vi "SetScanParameters.vi"(0 "Scan Parameters Cluster":T1={"Lines"=-2147483648, "Columns"=-2147483648, "X Range "=-inf, "Y Range "=-inf, "Pixel Size"=-inf, "Origin X"=-inf, "Origin Y"=-inf, "Rotation"=-inf, "Sample Time"=-inf} {"Sample Time" format="%#_g µs"; "Rotation" format="%#_g deg"; "Origin Y" format="%#_g nm"; "Origin X" format="%#_g nm"; "Pixel Size" format="%#_g nm"; "Y Range" format="%#_g nm"; "X Range" format="%#_g nm"; "Columns" max=250; "Lines" max=250}, 5 "error in":T3) -> (14 "Output Cluster":T1={"Lines"=-2147483648, "Columns"=-2147483648, "X Range "=-inf, "Y Range "=-inf, "Pixel Size"=-inf, "Origin X"=-inf, "Origin Y"=-inf, "Rotation"=-inf, "Sample Time"=-inf} {"Sample Time" format="%#_g µs"; "Rotation" format="%#_g deg"; "Origin Y" format="%#_g nm"; "Origin X" format="%#_g nm"; "Pixel Size" format="%#_g nm"; "Y Range" format="%#_g nm"; "X Range" format="%#_g nm"; "Columns" max=250; "Lines" max=250}, 19 "error out":T2)   [LabVIEW 2016]
doc: "Sets the parameters for a scan. Make sure to check if the chosen arguments are consistent with each other. The individual parts of the 'Scan Parameters Cluster' are:\n- Lines (integer) [0 to infinity]\n- Columns (integer) [0 to infinity]\n- Pixel Size (float) [0 to infinity]\n- Origin X (float) [0 to infinity]\n- Origin Y (float) [0 to infinity]\n- Rotation (float) [0 to infinity]\n- Sample Time (float) [0 to infinity]\n\n'Lines' and 'Columns' define the number of pixels the scan will have. The 'Pixel Size' states how large one single pixel will be. The 'Origin X' and 'Origin Y' parameters tell the controller where the field of scan shall be located. 'Rotation' fixes an angle by which the field is rotated. Every pixel will be measured with a certain time given by 'Sample Time'. By passing -Inf (float) or -2147483648 (integer) as input values, the corresponding parameter(s) will be read out."
uses:
  Controls/Scan_Parameters.ctl
  Controls/Error_In.ctl
  Controls/Error_Out.ctl
  Files_ASC500/DLL/ASC500_RemoteControlV27.dll
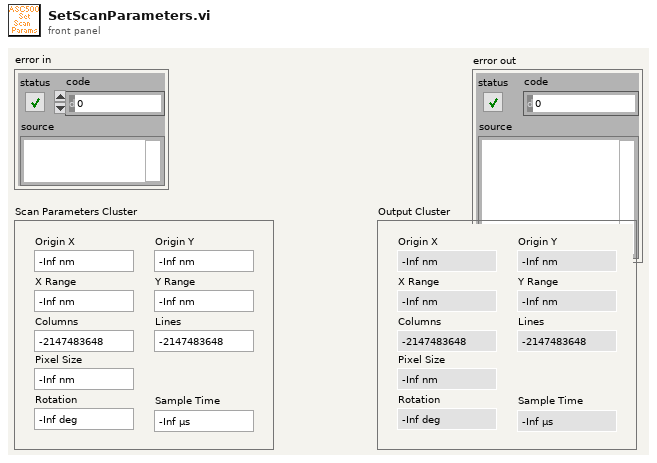
[diagram p1: front panel]
types:
  T1 = typedef "Scan_Parameters.ctl" = cluster{"Lines":i32, "Columns":i32, "X Range ":sgl, "Y Range ":sgl, "Pixel Size":sgl, "Origin X":sgl, "Origin Y":sgl, "Rotation":sgl, "Sample Time":sgl}
  T2 = typedef "Error_Out.ctl" = errorcluster
  T3 = typedef "Error_In.ctl" = errorcluster
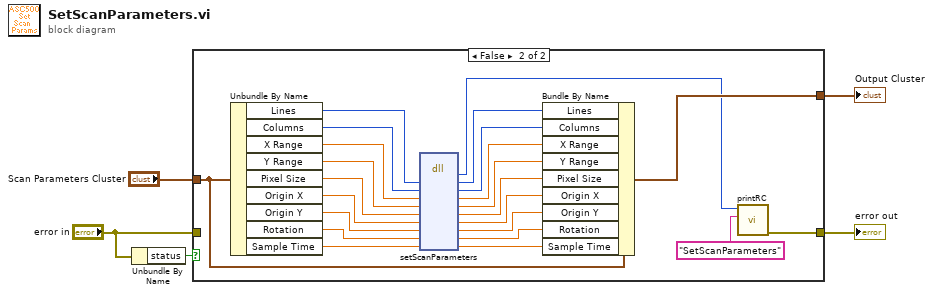
[diagram p0: block diagram]
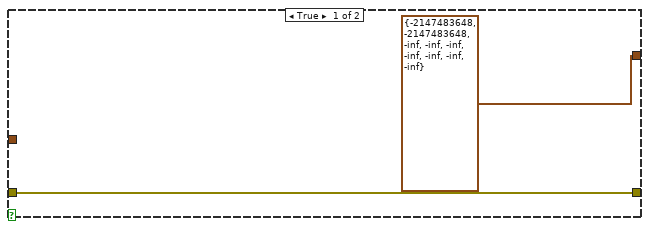
[diagram p2: hidden frame]
diagram:
  n1 = Unbundle By Name("error in") -> ("status"=w4:bool)
  n2 = case shown="False" w4 {
    tunnel: [w6 w10] -> w5
    tunnel: "Scan Parameters Cluster" -> [_ w15]
    tunnel: [T1 {"Lines"=-2147483648, "Columns"=-2147483648, "X Range "=-inf, "Y Range "=-inf, "Pixel Size"=-inf, "Origin X"=-inf, "Origin Y"=-inf, "Rotation"=-inf, "Sample Time"=-inf} ("Scan Parameters Cluster") w16] -> w2
    tunnel: "error in" -> [w6 _]
    frame True {
    }
    frame False {
      n3 = Unbundle By Name(w15) -> ("Lines"=w30:i32, "Columns"=w29:i32, "X Range"=w28:sgl, "Y Range"=w27:sgl, "Pixel Size"=w26:sgl, "Origin X"=w25:sgl, "Origin Y"=w24:sgl, "Rotation"=w13:sgl, "Sample Time"=w14:sgl)
      n4 = dll-call lib="G:/SCMOperations/Share/ELE/Produkt Information/ASC500/04 Remote Control/02 development versions/2018Nov06/Files_ASC500/DLL/ASC500_RemoteControlV27.dll" fn="setScanParameters"("Lines"=w30, "Columns"=w29, "X Range"=w28, "Y Range"=w27, "Pixel Size"=w26, "XOffset"=w25, "YOffset"=w24, "deg"=w13, "Sample Time"=w14) -> ("Rückgabetyp"=w9:i32, "Lines"=w23:i32, "Columns"=w22:i32, "X Range"=w21:sgl, "Y Range"=w20:sgl, "Pixel Size"=w19:sgl, "XOffset"=w18:sgl, "YOffset"=w17:sgl, "deg"=w11:sgl, "Sample Time"=w12:sgl)  [unwired: 3 in, 2 out]
      n5 = Bundle By Name(cluster=w15, "Lines"=w23, "Columns"=w22, "X Range"=w21, "Y Range"=w20, "Pixel Size"=w19, "Origin X"=w18, "Origin Y"=w17, "Rotation"=w11, "Sample Time"=w12) -> (w16:T1)
      n6 = call "printRC.vi"("additional information"="SetScanParameters", "RC"=w9) -> ("error out"=w10:T2)  [unwired: 9 in]
    }
  }
  "error out" <- w5
  "Output Cluster" <- w2
